vi "Leap POC.vi"() -> ()   [LabVIEW 2013]
uses:
  <vilib>/LabVIEW Hacker/Leap/Public/Gestures/Swipe/Instance VIs/Read 1 Swipe Direction.vi
  LVH-XBMC.lvlib
  Private/Type Defs/Input.Action.ctl
  <vilib>/LabVIEW Hacker/Leap/Private/Type Defs/Gesture State.ctl
panel:
  in  "Delay Between Events (ms)":u32
  out "Error Out":errorcluster
  in  "Stop Button":bool
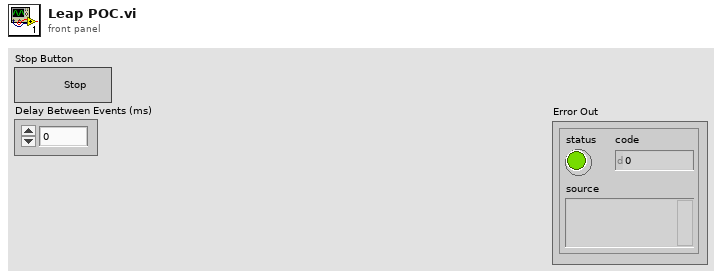
[diagram p1: front panel]
types:
  T1 = typedef "LVH-Leap.lvlib/Leap Handle.ctl" = cluster{"LeapCSharp":refnum<k24>}
  T2 = typedef "LVH-XBMC.lvlib/XBMC Ref.ctl" = cluster{"HTTP Handle":T3, "Hostname / IP":string, "jsonrpc":string}
  T3 = typedef "LabVIEWHTTPClient.lvlib/ClientHandle.ctl" = refnum<k1>
  T4 = typedef "LVH-Leap.lvlib/Gesture State.ctl" = enum16{"Invalid", "Start", "Update", "Stop"}
  T5 = typedef "LVH-XBMC.lvlib/Input.Action.ctl" = enum16{"left", "right", "up", "down", "pageup", "pagedown", "select", "highlight", "parentdir", "parentfolder", "back", "previousmenu", "info", "pause", "stop", "skipnext", "skipprevious", "fullscreen", "aspectratio", "stepforward", "stepback", "bigstepforward", "bigstepback", "chapterorbigstepforward", "chapterorbigstepback", "osd", "showsubtitles", "nextsubtitle", "codecinfo", "nextpicture", "previouspicture", "zoomout", "zoomin", "playlist", "queue", "zoomnormal", "zoomlevel1", "zoomlevel2", "zoomlevel3", "zoomlevel4", "zoomlevel5", "zoomlevel6", "zoomlevel7", "zoomlevel8", "zoomlevel9", "nextcalibration", "resetcalibration", "analogmove", "rotate", "rotateccw", "close", "subtitledelayminus", "subtitledelay", "subtitledelayplus", "audiodelayminus", "audiodelay", "audiodelayplus", "subtitleshiftup", "subtitleshiftdown", "subtitlealign", "audionextlanguage", "verticalshiftup", "verticalshiftdown", "nextresolution", "audiotoggledigital", "number0", "number1", "number2", "number3", "number4", "number5", "number6", "number7", "number8", "number9", "osdleft", "osdright", "osdup", "osddown", "osdselect", "osdvalueplus", "osdvalueminus", "smallstepback", "fastforward", "rewind", "play", "playpause", "switchplayer", "delete", "copy", "move", "mplayerosd", "hidesubmenu", "screenshot", "rename", "togglewatched", "scanitem", "reloadkeymaps", "volumeup", "volumedown", "mute", "backspace", "scrollup", "scrolldown", "analogfastforward", "analogrewind", "moveitemup", "moveitemdown", "contextmenu", "shift", "symbols", "cursorleft", "cursorright", "showtime", "analogseekforward", "analogseekback", "showpreset", "presetlist", "nextpreset", "previouspreset", "lockpreset", "randompreset", "increasevisrating", "decreasevisrating", "showvideomenu", "enter", "increaserating", "decreaserating", "togglefullscreen", "nextscene", "previousscene", "nextletter", "prevletter", "jumpsms2", "jumpsms3", "jumpsms4", "jumpsms5", "jumpsms6", "jumpsms7", "jumpsms8", "jumpsms9", "filter", "filterclear", "filtersms2", "filtersms3", "filtersms4", "filtersms5", "filtersms6", "filtersms7", "filtersms8", "filtersms9", "firstpage", "lastpage", "guiprofile", "red", "green", "yellow", "blue", "increasepar", "decreasepar", "volampup", "volampdown", "createbookmark", "createepisodebookmark", "settingsreset", "settingslevelchange", "stereomode", "nextstereomode", "previousstereomode", "togglestereomode", "stereomodetomono", "channelup", "channeldown", "previouschannelgroup", "nextchannelgroup", "playpvr", "playpvrtv", "playpvrradio", "record", "leftclick", "rightclick", "middleclick", "doubleclick", "wheelup", "wheeldown", "mousedrag", "mousemove", "tap", "longpress", "pangesture", "zoomgesture", "rotategesture", "swipeleft", "swiperight", "swipeup", "swipedown", "noop"}
  T6 = typedef "LVH-Leap.lvlib/Swipe Direction.ctl" = enum16{"Left", "Right", "Up", "Down", "In", "Out"}
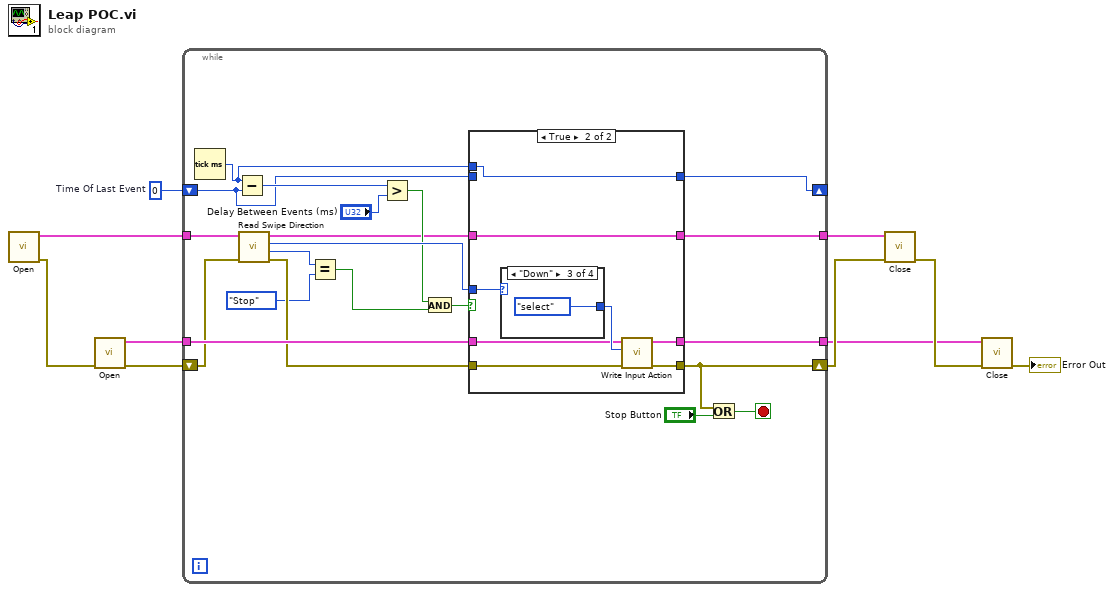
[diagram p0: block diagram]
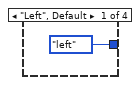
[diagram p3: hidden frame]
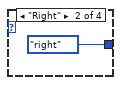
[diagram p4: hidden frame]
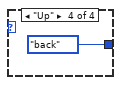
[diagram p5: hidden frame]
diagram:
  w1 = u32 0  # Time Of Last Event
  n1 = call <vilib>:"Open.vi"() -> ("Error Out"=w7:errorcluster, "Leap Handle"=w10:T1)  [unwired: 10 in]
  n2 = call <vilib>:"Open.vi"("Error In"=w7) -> ("Error Out"=w8:errorcluster, "XBMC Ref"=w9:T2)  [unwired: 9 in]
  n3 = while {
    tunnel: w10 -> [w11]
    tunnel: w9 -> [w28]
    tunnel: [w25] -> w3
    tunnel: [w15] -> w2
    shift-right: [w24] -> w6
    shift-left: w8 -> [w27]
    shift-right: [w12] -> _
    shift-left: w1 -> [w13]
    stop <- w31 stop-if-true
    n4 = Tick Count (ms)() -> (millisecond timer value=w14:u32)
    n5 = Subtract(x=w14, y=w13) -> (x-y=w23:u32)
    n6 = call-poly <vilib>:"Read Swipe Direction.vi"("Error In"=w27, "Leap Handle"=w11) -> ("Error Out"=w26:errorcluster, "Gesture State"=w21:T4, "Swipe Direction"=w29:T6, "Leap Handle"=w16:T1)  [unwired: 6 in]
    n7 = Equal?(x=w21, y=Gesture_State."Stop") -> (x = y?=w18:bool)
    n8 = Greater?(x=w23, y="Delay Between Events (ms)") -> (0:w19:bool)
    n9 = And(x=w19, y=w18) -> (x .and. y?=w17:bool)
    n10 = case shown="True" w17 {
      tunnel: w29 -> [_ w43]
      tunnel: w28 -> [w35 w41]
      tunnel: w26 -> [w34 w40]
      tunnel: [w34 w39] -> w24
      tunnel: [w35 w38] -> w25
      tunnel: w16 -> [w33 w37]
      tunnel: [w33 w37] -> w15
      tunnel: w14 -> [_ w36]
      tunnel: w13 -> [w32 _]
      tunnel: [w32 w36] -> w12
      frame False {
      }
      frame True {
        n11 = case shown="\"Down\"" w43 {
          tunnel: [Input.Action."left" ("Input Action") Input.Action."right" ("Input Action") Input.Action."select" ("Input Action") Input.Action."back" ("Input Action")] -> w42
          frame "Left", Default {
          }
          frame "Right" {
          }
          frame "Down" {
          }
          frame "Up" {
          }
        }
        n12 = call "Write Input Action.vi"("Error In"=w40, "Input Action"=w42, "XBMC Ref"=w41) -> ("Error Out"=w39:errorcluster, "XBMC Ref"=w38:T2)  [unwired: 7 in]
      }
    }
    n13 = Or(x=w24, y="Stop Button") -> (x .or. y?=w31:bool)
  }
  n14 = call <vilib>:"Close.vi"("Error In"=w6, "Leap Handle"=w2) -> ("Error Out"=w4:errorcluster)  [unwired: 9 in]
  n15 = call <vilib>:"Close.vi"("Error In"=w4, "XBMC Ref"=w3) -> ("Error Out"=→"Error Out":errorcluster)  [unwired: 9 in]
